vi "FPGA_Constants.vi"() -> (0 "Sampling Rate":fxp<+,30,25>=26666666.59375, 1 "Time Out Limit":fxp<+,21,-8>=0.0034999996423721313)   [LabVIEW 2015]
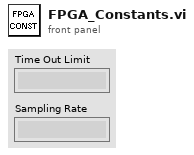
[diagram p1: front panel]
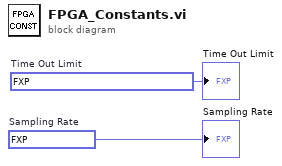
[diagram p0: block diagram]
diagram:
  w1 = fxp<+,30,25> 26666666.59375  # Sampling Rate
  w2 = fxp<+,21,-8> 0.0034999996423721313  # Time Out Limit
  "Time Out Limit" <- w2
  "Sampling Rate" <- w1
